vi "Read Frequency Domain Measurement Data.vi"(8 "error in (no error)":errorcluster, 11 "VISA resource name":refnum<visa-resource-name>) -> (0 "error out":errorcluster, 1 "Channel Power":dbl, 2 "Measurement Type":u16(ring) items=["None", "Channel Power", "Adjacent Channel Power Ratio", "Occupied Bandwidth"], 3 "VISA resource name out":refnum<visa-resource-name>, 5 "Units":u16(ring) items=["dBm", "dBµW", "dBmV", "dbµV", "dbmA", "dBµA"])   [LabVIEW 2010, in "Tektronix DPO MSO 2000 4000 Series.lvlib"]
doc: "Returns the Measurement Type and the Channel Power for the Frequency Domain Measurement configured for the MDO series oscilloscope."
uses:
  <instrlib>/Tektronix DPO MSO 2000 4000 Series/Tektronix DPO MSO 2000 4000 Series.lvlib
  <vilib>/regexp/Match Regular Expression.xnode
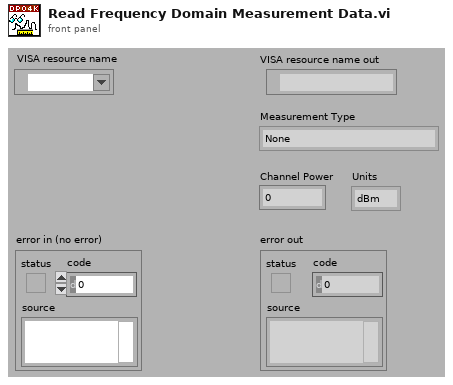
[diagram p1: front panel]
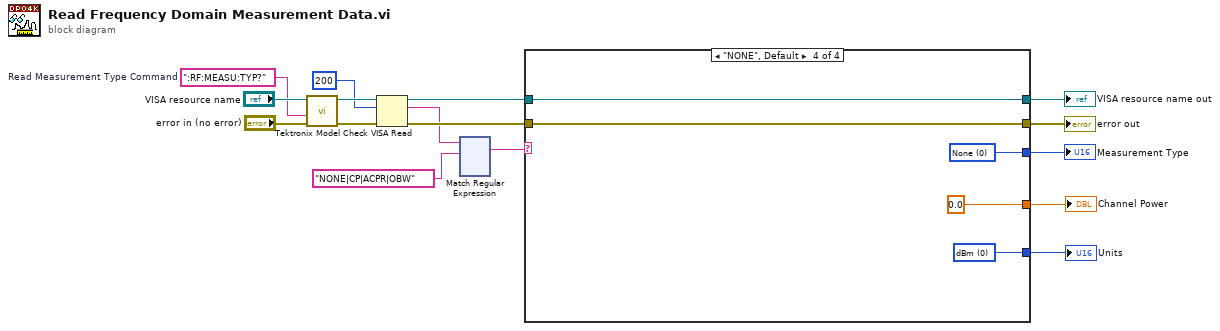
[diagram p0: block diagram]
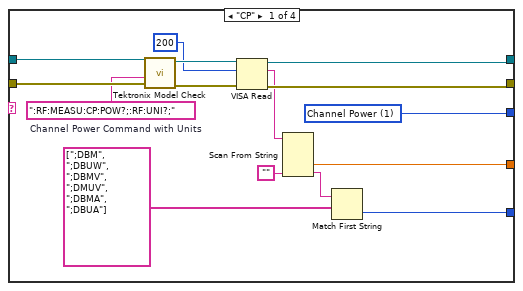
[diagram p2: hidden frame]
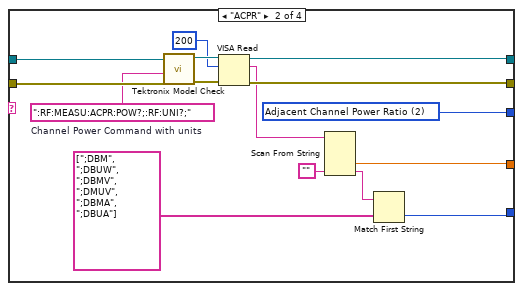
[diagram p3: hidden frame]
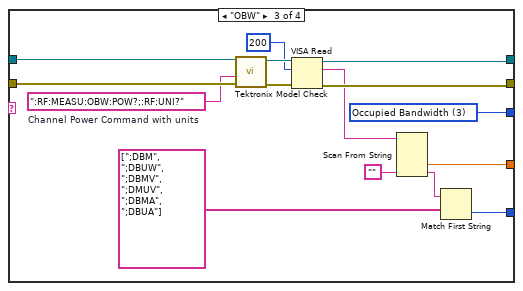
[diagram p4: hidden frame]
diagram:
  w14 = ":RF:MEASU:TYP?"  # Read Measurement Type Command
  n1 = call <instrlib>:"Tektronix Model Check.vi"("error in (no error)"="error in (no error)", "Command String"=w14, "VISA resource name"="VISA resource name") -> ("error out"=w12:errorcluster, "VISA resource name out"=w13:refnum<visa-resource-name>)  [unwired: 7 in]
  n2 = VISA Read(VISA resource name=w13, byte count=u32 200, error in (no error)=w12) -> (VISA resource name out=w10:refnum<visa-resource-name>, read buffer=w3:string, error out=w9:errorcluster)  [unwired: 1 out]
  n3 = xnode "Match Regular Expression"("input string"=w3, "regular expression"="NONE|CP|ACPR|OBW") -> ("whole match"=w2:string)  [unwired: 4 in, 4 out]
  n4 = case shown="\"NONE\", Default" w2 {
    tunnel: w10 -> [w31 w46 w61 w66]
    tunnel: w9 -> [w30 w45 w60 w65]
    tunnel: [w24 w38 w54 w66] -> w8
    tunnel: [w23 w37 w53 w65] -> w7
    tunnel: [w28 w39 w52 w64] -> w6
    tunnel: [w22 w40 w55 0.0 ("Channel Power")] -> w5
    tunnel: [w19 w34 w49 w62] -> w1
    frame "CP" {
      w28 = u16 1 items=["None", "Channel Power", "Adjacent Channel Power Ratio", "Occupied Bandwidth"] ("Measurement Type")
      w29 = ":RF:MEASU:CP:POW?;:RF:UNI?;"  # Channel Power Command with Units
      n5 = call <instrlib>:"Tektronix Model Check.vi"("error in (no error)"=w30, "Command String"=w29, "VISA resource name"=w31) -> ("error out"=w26:errorcluster, "VISA resource name out"=w27:refnum<visa-resource-name>)  [unwired: 7 in]
      n6 = VISA Read(VISA resource name=w27, byte count=u32 200, error in (no error)=w26) -> (VISA resource name out=w24:refnum<visa-resource-name>, read buffer=w20:string, error out=w23:errorcluster)  [unwired: 1 out]
      n7 = Scan From String(input string=w20, default 2="") -> (output 1=w22:dbl, output 2=w17:string)  [unwired: 4 in, 3 out]
      n8 = Match First String(2:string[] [";DBM", ";DBUW", ";DBMV", ";DMUV", ";DBMA", ";DBUA"] ("string array"), 3:w17) -> (0:w19:i32)  [unwired: 1 out]
    }
    frame "ACPR" {
      w39 = u16 2 items=["None", "Channel Power", "Adjacent Channel Power Ratio", "Occupied Bandwidth"] ("Measurement Type")
      w44 = ":RF:MEASU:ACPR:POW?;:RF:UNI?;"  # Channel Power Command with units
      n9 = call <instrlib>:"Tektronix Model Check.vi"("error in (no error)"=w45, "Command String"=w44, "VISA resource name"=w46) -> ("error out"=w42:errorcluster, "VISA resource name out"=w43:refnum<visa-resource-name>)  [unwired: 7 in]
      n10 = VISA Read(VISA resource name=w43, byte count=u32 200, error in (no error)=w42) -> (VISA resource name out=w38:refnum<visa-resource-name>, read buffer=w35:string, error out=w37:errorcluster)  [unwired: 1 out]
      n11 = Scan From String(input string=w35, default 2="") -> (output 1=w40:dbl, output 2=w32:string)  [unwired: 4 in, 3 out]
      n12 = Match First String(2:string[] [";DBM", ";DBUW", ";DBMV", ";DMUV", ";DBMA", ";DBUA"] ("string array"), 3:w32) -> (0:w34:i32)  [unwired: 1 out]
    }
    frame "OBW" {
      w52 = u16 3 items=["None", "Channel Power", "Adjacent Channel Power Ratio", "Occupied Bandwidth"] ("Measurement Type")
      w59 = ":RF:MEASU:OBW:POW?;:RF:UNI?"  # Channel Power Command with units
      n13 = call <instrlib>:"Tektronix Model Check.vi"("error in (no error)"=w60, "Command String"=w59, "VISA resource name"=w61) -> ("error out"=w58:errorcluster, "VISA resource name out"=w57:refnum<visa-resource-name>)  [unwired: 7 in]
      n14 = VISA Read(VISA resource name=w57, byte count=u32 200, error in (no error)=w58) -> (VISA resource name out=w54:refnum<visa-resource-name>, read buffer=w50:string, error out=w53:errorcluster)  [unwired: 1 out]
      n15 = Scan From String(input string=w50, default 2="") -> (output 1=w55:dbl, output 2=w47:string)  [unwired: 4 in, 3 out]
      n16 = Match First String(2:string[] [";DBM", ";DBUW", ";DBMV", ";DMUV", ";DBMA", ";DBUA"] ("string array"), 3:w47) -> (0:w49:i32)  [unwired: 1 out]
    }
    frame "NONE", Default {
      w62 = u16 0 items=["dBm", "dBµW", "dBmV", "dbµV", "dbmA", "dBµA"] ("Units")
      w64 = u16 0 items=["None", "Channel Power", "Adjacent Channel Power Ratio", "Occupied Bandwidth"] ("Measurement Type")
    }
  }
  "error out" <- w7
  "VISA resource name out" <- w8
  "Measurement Type" <- w6
  "Channel Power" <- w5
  "Units" <- w1
